vi "Get All Property.vi"(8 "error in":errorcluster, 11 "Item in":refnum<class "Item.lvclass">) -> (0 "error out":errorcluster, 3 "Properties out":refnum<class "Property.lvclass">[](array[class]))   [LabVIEW 2024, in "Parser.lvlib" / "Property.lvclass"]
uses:
  Property.lvclass
  Property.lvclass/Property.ctl
  Item/Item.lvclass
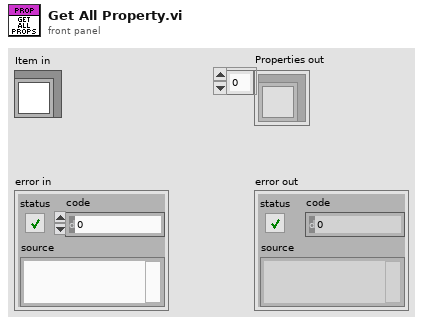
[diagram p1: front panel]
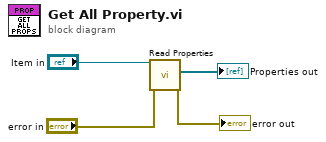
[diagram p0: block diagram]
diagram:
  n1 = call "Read Properties.vi"("error in"="error in", "Item in"="Item in") -> ("error out"=→"error out":errorcluster, "Properties"=→"Properties out":refnum<class "Property.lvclass">[])  [unwired: 7 in, 1 out]
